vi "Gen Modbus Test.vi"() -> ()   [LabVIEW 2014]
uses:
  Controls/Gen Data.ctl
  Controls/NamedError.ctl
panel:
  out "Gen West Error 2":T1
  out "Gen West Count 2":i32
  in  "Clear Error 2":bool
  out "Generator ON West 2":bool=TRUE
  out "Generator ON East 2":bool=TRUE
  in  "stop 2":bool
  out "Gen Data 2":T2 {"TotalFuel(L)" format="%.2f"; "FuelRate(L/H)" format="%.2f"; "ApparentPower(VA)" format="%.2f"; "BattVoltage(V)" format="%.2f"; "Freq(Hz)" format="%.2f"; "RunHours(hr)" format="%.2f"; "PowerFactor" format="%.2f"; "ReactivePower(VAR)" format="%.2f"; "ActivePower(W)" format="%.2f"}
  out "Gen Data":T2 {"TotalFuel(L)" format="%.2f"; "FuelRate(L/H)" format="%.2f"; "ApparentPower(VA)" format="%.2f"; "BattVoltage(V)" format="%.2f"; "Freq(Hz)" format="%.2f"; "RunHours(hr)" format="%.2f"; "PowerFactor" format="%.2f"; "ReactivePower(VAR)" format="%.2f"; "ActivePower(W)" format="%.2f"}
  out "Generator ON East":bool=TRUE
  out "Generator ON West":bool=TRUE
  out "Gen West Error":T1
  out "Gen West Count":i32
  in  "Clear Error":bool
  in  "stop":bool
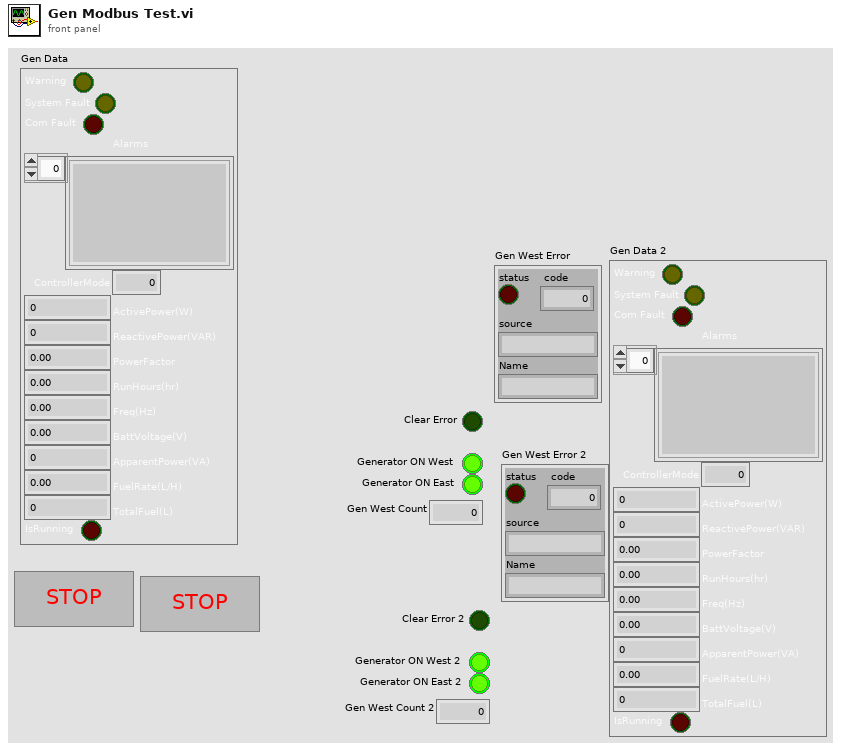
[diagram p1: front panel]
types:
  T1 = typedef "NamedError.ctl" = cluster{"status":bool, "code":i32, "source":string, "Name":string}
  T2 = typedef "Gen Data.ctl" = cluster{"Warning":bool, "System Fault":bool, "Com Fault":bool, "Alarms":string[], "ControllerMode":u16, "ActivePower(W)":i32, "ReactivePower(VAR)":i32, "PowerFactor":dbl, "RunHours(hr)":dbl, "Freq(Hz)":dbl, "BattVoltage(V)":dbl, "ApparentPower(VA)":i32, "FuelRate(L/H)":dbl, "TotalFuel(L)":u32, "IsRunning":bool}
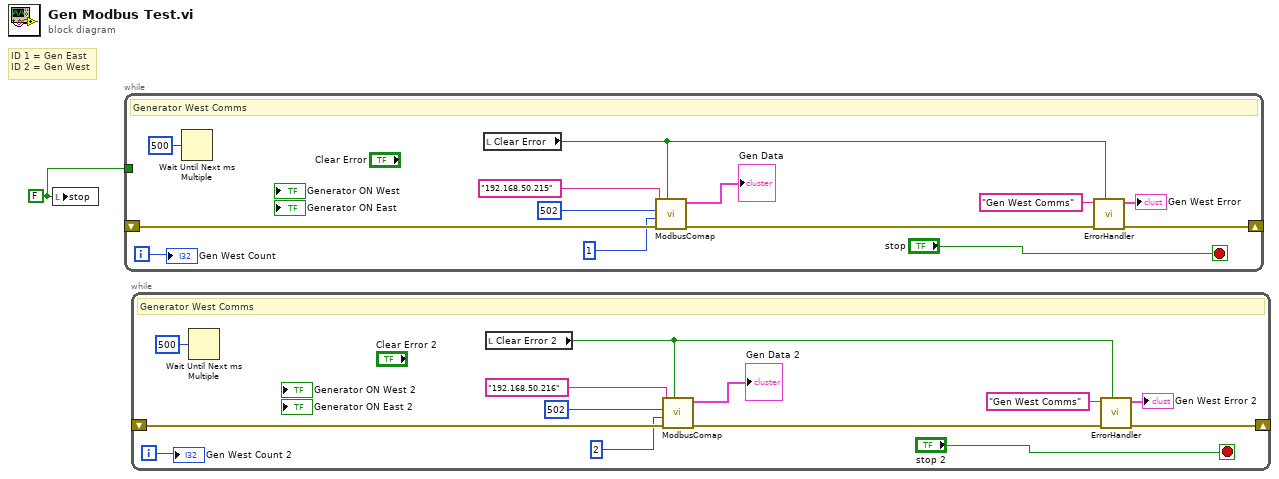
[diagram p0: block diagram]
diagram:
  w1 = FALSE ("stop")
  # "ID 1 = Gen East\nID 2 = Gen West"
  n1 = local write "stop"(w1) -> ()
  n2 = while "Generator Comms" {
    shift-right: [w11] -> _
    shift-left: _ -> [w5]
    tunnel: w1 -> [_]
    i -> [w6]
    stop <- "stop" stop-if-true
    # "Generator West Comms"
    n3 = Wait Until Next ms Multiple(millisecond multiple=u32 500 ("milliseconds to wait")) -> ()  [unwired: 1 out]
    n4 = local read "Clear Error"() -> (w7:bool)
    n5 = call "ModbusComap.vi"("address"="192.168.50.215", "port (502)"=u16 502, "Unit ID"=u8 1, "Error In"=w5, 4:w7) -> ("Gen Data"=→"Gen Data":T2, "Error Out"=w10:errorcluster)  [unwired: 4 in]
    n6 = call "ErrorHandler.vi"("Clear Error"=w7, "Error In"=w10, "Name"="Gen West Comms") -> ("Error Out"=w11:errorcluster, "Named Error Out"=→"Gen West Error":T1)  [unwired: 5 in]
    "Gen West Count" <- w6
  }
  n7 = while "Generator Comms" {
    shift-right: [w24] -> _
    shift-left: _ -> [w18]
    i -> [w19]
    stop <- "stop 2" stop-if-true
    # "Generator West Comms"
    n8 = Wait Until Next ms Multiple(millisecond multiple=u32 500 ("milliseconds to wait")) -> ()  [unwired: 1 out]
    n9 = local read "Clear Error 2"() -> (w20:bool)
    n10 = call "ModbusComap.vi"("address"="192.168.50.216", "port (502)"=u16 502, "Unit ID"=u8 2, "Error In"=w18, 4:w20) -> ("Gen Data"=→"Gen Data 2":T2, "Error Out"=w23:errorcluster)  [unwired: 4 in]
    n11 = call "ErrorHandler.vi"("Clear Error"=w20, "Error In"=w23, "Name"="Gen West Comms") -> ("Error Out"=w24:errorcluster, "Named Error Out"=→"Gen West Error 2":T1)  [unwired: 5 in]
    "Gen West Count 2" <- w19
  }
